vi "Test AO.vi"() -> ()   [LabVIEW 2009, in "MicroDAQ.lvlib"]
uses:
  <instrlib>/MicroDAQ/MicroDAQ.lvlib
  <instrlib>/MicroDAQ/Temp Tests/Test AO enum.ctl
  <instrlib>/MicroDAQ/Tools/Analog mode.ctl
  <instrlib>/MicroDAQ/Tools/Analog Channel Enum.ctl
  <instrlib>/MicroDAQ/Tools/Analo Range Enum.ctl
  <instrlib>/MicroDAQ/Channel/Analog Output/Write NChan NSamp 2D SGL.vi
  <instrlib>/MicroDAQ/Channel/Analog Output/AO Configure Channel.vi
  <instrlib>/MicroDAQ/Channel/Analog Output/Analog output.lvclass
  <instrlib>/MicroDAQ/Channel/Analog Output/Write 1Chan 1Sample SGL.vi
  <instrlib>/MicroDAQ/Channel/Analog Output/Write NChan 1Sample 1D SGL.vi
  <instrlib>/MicroDAQ/MLink32.dll
panel:
  out "Current Test":T1
  in  "Test to execute":T1[](array[typedef])=[enum."Default Config Write NChan NSamp", enum."Default Config Write 1Chan 1Sample", enum."Default Config Write 1Chan 1Sample (with Start)"]
  out "error occured":errorcluster
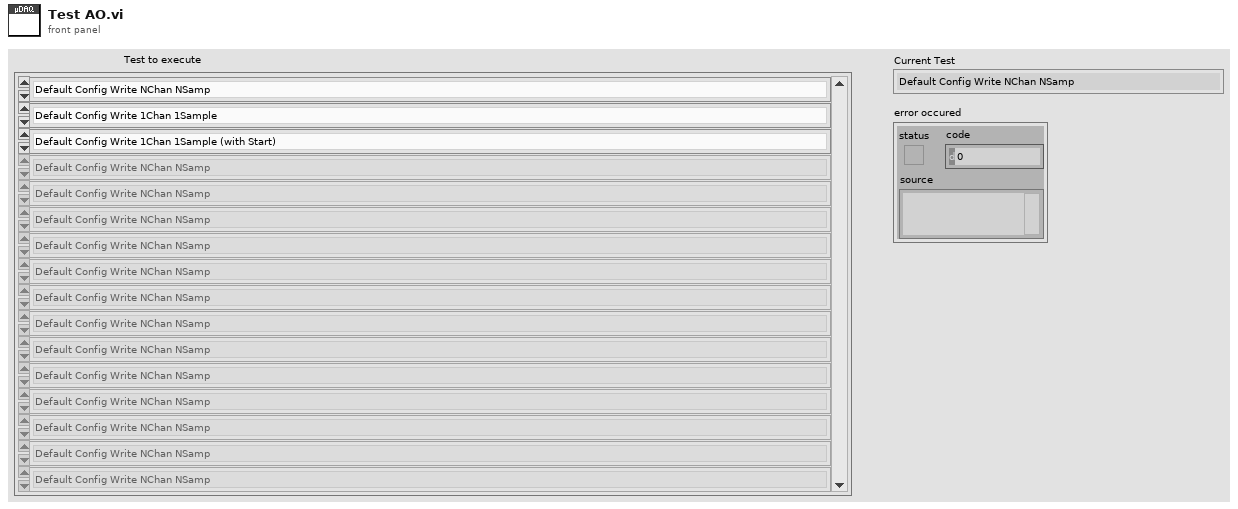
[diagram p1: front panel]
types:
  T1 = typedef "MicroDAQ.lvlib/Test AO enum.ctl" = enum16{"Default Config Write NChan NSamp", "Default Config Write 1Chan 1Sample", "Default Config Write 1Chan 1Sample (with Start)", "Default Config 2Chan NSamp followed by Write 1Samp", "Default Config 2Chan NSamp followed by Write 1Samp followed by Write NSamp"}
  T2 = typedef "MicroDAQ.lvlib/Analog mode.ctl" = enum16{"Periodic", "Stream"}
  T3 = typedef "MicroDAQ.lvlib/Analog Channel Enum.ctl" = enum16{"None", "AO1", "AO2", "AO3", "AO4", "AO5", "AO6", "AO7", "AO8", "AO9", "AO10", "AO11", "AO12", "AO13", "AO14", "AO15", "AO16"}
  T4 = typedef "MicroDAQ.lvlib/Analo Range Enum.ctl" = enum16{"±10V", "0-10V", "±5V", "0-5V", "±5.12V", "±2.56V", "±2.5V", "±2V", "±1.24V", "±0.64V"}
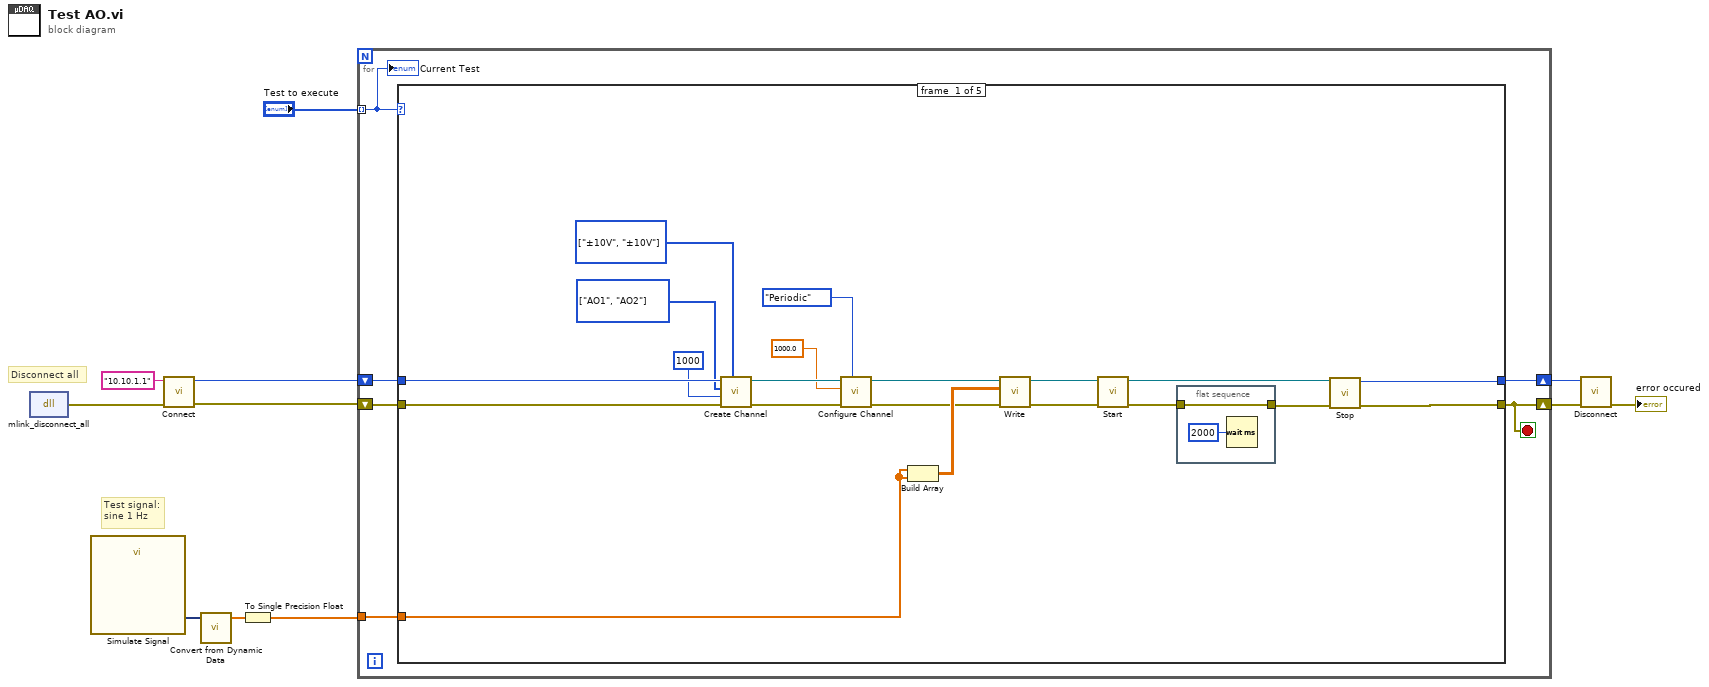
[diagram p0: block diagram]
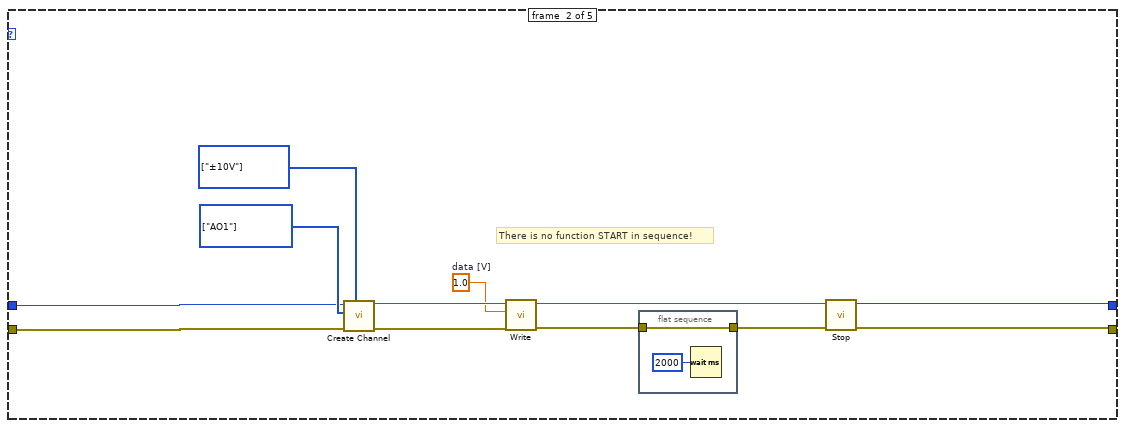
[diagram p2: hidden frame]
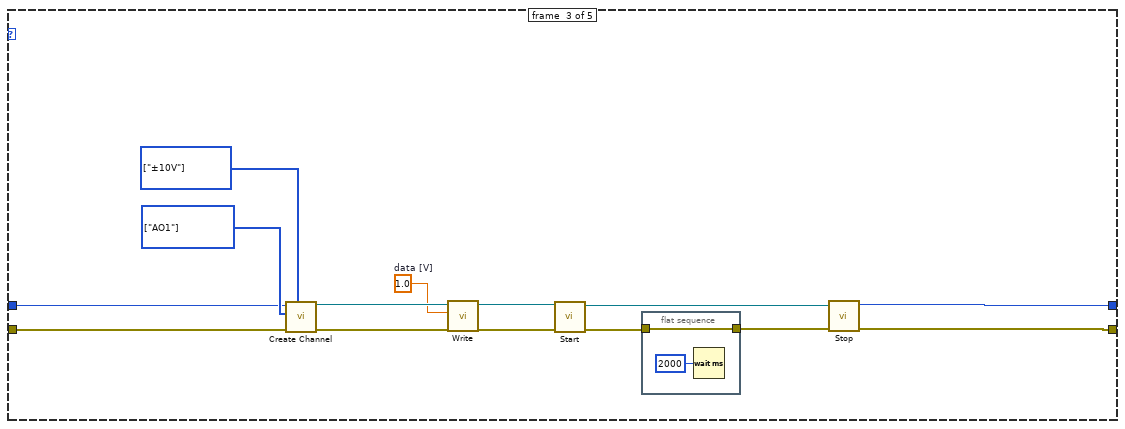
[diagram p3: hidden frame]
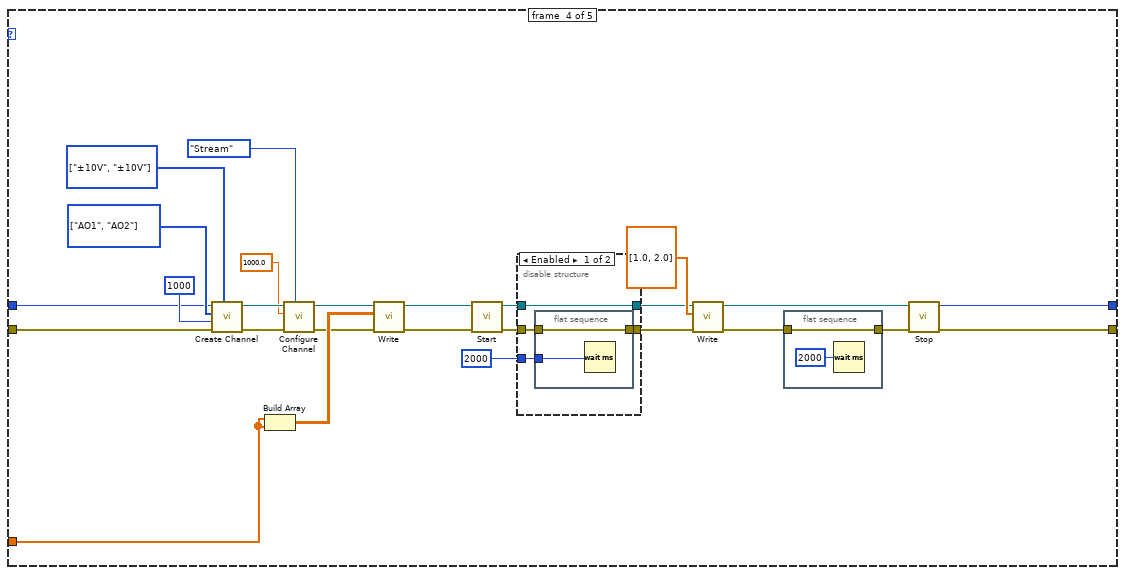
[diagram p4: hidden frame]
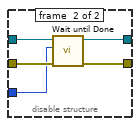
[diagram p5: hidden frame]
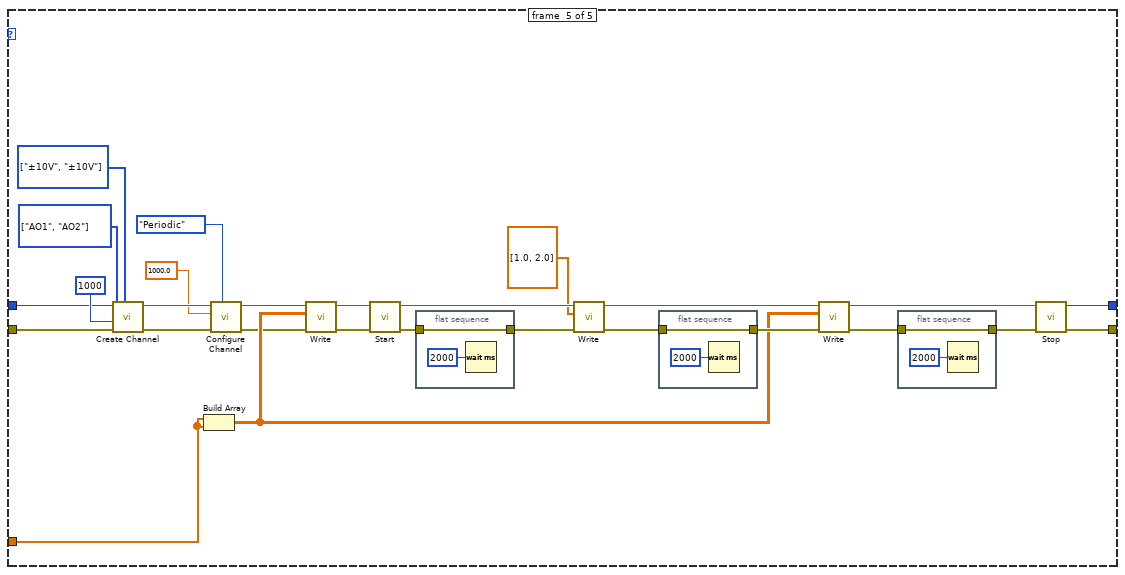
[diagram p6: hidden frame]
diagram:
  # "Test signal:\nsine 1 Hz"
  # "Disconnect all"
  n1 = dll-call lib="C:/Program Files (x86)/National Instruments/LabVIEW 2009/instr.lib/MicroDAQ/MLink32.dll" fn="mlink_disconnect_all" ("MLink32.*:mlink_connect")() -> (error out=w11:errorcluster)  [unwired: 4 in, 1 out]
  n2 = call "Simulate Signal"() -> ("Sine"=w7:dynamicdata)  [unwired: 14 in, 1 out]
  n3 = call <instrlib>:"Connect.vi"("error in (no error)"=w11, "IP address"="10.10.1.1") -> ("error out"=w9:errorcluster, "connection ID"=w10:i32)  [unwired: 8 in]
  n4 = call "Convert from Dynamic Data"("Dynamic Data Type"=w7) -> ("Array"=w6:dbl[])  [unwired: 3 in]
  n5 = To Single Precision Float(number=w6) -> (single precision float=w5:sgl[])
  n6 = for {
    tunnel: w5 -> [w15]
    tunnel: "Test to execute" -> [w14] mode=indexing
    shift-right: [w13] -> w3
    shift-left: w10 -> [w17]
    shift-right: [w12] -> w2
    shift-left: w9 -> [w16]
    stop <- w12 stop-if-true
    n7 = case shown="\"Default Config 2Chan NSamp followed by Write 1Samp followed by Write NSamp\"" w14 {
      tunnel: w17 -> [w37 w49 w61 w80 w125]
      tunnel: w16 -> [w36 w48 w60 w79 w124]
      tunnel: w15 -> [w31 _ _ w83 w123]
      tunnel: [w25 w41 w58 w85 w118] -> w12
      tunnel: [w24 w40 w59 w84 w119] -> w13
      frame #0 {
        w34 = T3[] [enum."AO1", enum."AO2"] items=["None", "AO1", "AO2", "AO3", "AO4", "AO5", "AO6", "AO7", "AO8", "AO9", "AO10", "AO11", "AO12", "AO13", "AO14", "AO15", "AO16"] ("channels")
        w35 = T4[] [enum."±10V", enum."±10V"] items=["±10V", "0-10V", "±5V", "0-5V", "±5.12V", "±2.56V", "±2.5V", "±2V", "±1.24V", "±0.64V"] ("ranges")
        # "AO Basic Config Write (2s) test, 2 Channels"
        n8 = call-poly <instrlib>:"Create Channel.vi"("Ranges"=w35, "error in (no error)"=w36, "Buffer size"=1000 ("buffor size"), "Phisical channels"=w34, "Connection ID"=w37) -> ("error out"=w21:errorcluster, "Task Out"=w23:refnum<class "Analog output.lvclass">)  [unwired: 5 in]
        n9 = call-poly <instrlib>:"Configure Channel.vi"("Mode"=Analog_mode."Periodic", "error in (no error)"=w21, "Sample rate"=1000.0, "Analog Output in"=w23) -> ("error out"=w20:errorcluster, "Analog Output out"=w19:refnum<class "Analog output.lvclass">)  [unwired: 6 in]
        n10 = Build Array(w31, w31) -> (w32:sgl[][])
        n11 = call-poly <instrlib>:"Write.vi"("error in (no error)"=w20, "data"=w32, "Analog Output in"=w19) -> ("error out"=w29:errorcluster, "Analog Output out"=w30:refnum<class "Analog output.lvclass">)  [unwired: 7 in]
        n12 = call-dynamic "Start.vi"("error in (no error)"=w29, "Analog Output in"=w30) -> ("error out"=w28:errorcluster, "Analog Output out"=w26:refnum<class "Analog output.lvclass">)  [unwired: 8 in]
        n13 = flat-sequence {
          tunnel: w28 -> [w38]
          tunnel: [w38] -> w27
          frame #0 {
            n14 = Wait (ms)(milliseconds to wait=u32 2000) -> ()  [unwired: 1 out]
          }
        }
        n15 = call-dynamic "Stop.vi"("error in (no error)"=w27, "Analog Output in"=w26) -> ("error out"=w25:errorcluster, "connection ID"=w24:i32)  [unwired: 8 in]
      }
      frame #1 {
        w45 = sgl 1.0  # data [V]
        w50 = T3[] [enum."AO1"] items=["None", "AO1", "AO2", "AO3", "AO4", "AO5", "AO6", "AO7", "AO8", "AO9", "AO10", "AO11", "AO12", "AO13", "AO14", "AO15", "AO16"] ("channels")
        w51 = T4[] [enum."±10V"] items=["±10V", "0-10V", "±5V", "0-5V", "±5.12V", "±2.56V", "±2.5V", "±2V", "±1.24V", "±0.64V"] ("ranges")
        # "There is no function START in sequence!"
        n16 = call-poly <instrlib>:"Create Channel.vi"("Ranges"=w51, "error in (no error)"=w48, "Phisical channels"=w50, "Connection ID"=w49) -> ("error out"=w46:errorcluster, "Task Out"=w47:refnum<class "Analog output.lvclass">)  [unwired: 6 in]
        n17 = call-poly <instrlib>:"Write.vi"("error in (no error)"=w46, "data"=w45, "Analog Output in"=w47) -> ("error out"=w43:errorcluster, "Analog Output out"=w44:refnum<class "Analog output.lvclass">)  [unwired: 7 in]
        n18 = flat-sequence {
          tunnel: w43 -> [w52]
          tunnel: [w52] -> w42
          frame #0 {
            n19 = Wait (ms)(milliseconds to wait=u32 2000) -> ()  [unwired: 1 out]
          }
        }
        n20 = call-dynamic "Stop.vi"("error in (no error)"=w42, "Analog Output in"=w44) -> ("error out"=w41:errorcluster, "connection ID"=w40:i32)  [unwired: 8 in]
      }
      frame #2 {
        w63 = sgl 1.0  # data [V]
        w66 = T3[] [enum."AO1"] items=["None", "AO1", "AO2", "AO3", "AO4", "AO5", "AO6", "AO7", "AO8", "AO9", "AO10", "AO11", "AO12", "AO13", "AO14", "AO15", "AO16"] ("channels")
        w67 = T4[] [enum."±10V"] items=["±10V", "0-10V", "±5V", "0-5V", "±5.12V", "±2.56V", "±2.5V", "±2V", "±1.24V", "±0.64V"] ("ranges")
        n21 = call-poly <instrlib>:"Create Channel.vi"("Ranges"=w67, "error in (no error)"=w60, "Phisical channels"=w66, "Connection ID"=w61) -> ("error out"=w64:errorcluster, "Task Out"=w65:refnum<class "Analog output.lvclass">)  [unwired: 6 in]
        n22 = call-poly <instrlib>:"Write.vi"("error in (no error)"=w64, "data"=w63, "Analog Output in"=w65) -> ("error out"=w57:errorcluster, "Analog Output out"=w56:refnum<class "Analog output.lvclass">)  [unwired: 7 in]
        n23 = call-dynamic "Start.vi"("error in (no error)"=w57, "Analog Output in"=w56) -> ("error out"=w54:errorcluster, "Analog Output out"=w55:refnum<class "Analog output.lvclass">)  [unwired: 8 in]
        n24 = flat-sequence {
          tunnel: w54 -> [w68]
          tunnel: [w68] -> w62
          frame #0 {
            n25 = Wait (ms)(milliseconds to wait=u32 2000) -> ()  [unwired: 1 out]
          }
        }
        n26 = call-dynamic "Stop.vi"("error in (no error)"=w62, "Analog Output in"=w55) -> ("error out"=w58:errorcluster, "connection ID"=w59:i32)  [unwired: 8 in]
      }
      frame #3 {
        w94 = T3[] [enum."AO1", enum."AO2"] items=["None", "AO1", "AO2", "AO3", "AO4", "AO5", "AO6", "AO7", "AO8", "AO9", "AO10", "AO11", "AO12", "AO13", "AO14", "AO15", "AO16"] ("channels")
        w95 = T4[] [enum."±10V", enum."±10V"] items=["±10V", "0-10V", "±5V", "0-5V", "±5.12V", "±2.56V", "±2.5V", "±2V", "±1.24V", "±0.64V"] ("ranges")
        n27 = call-poly <instrlib>:"Create Channel.vi"("Ranges"=w95, "error in (no error)"=w79, "Buffer size"=1000 ("buffor size"), "Phisical channels"=w94, "Connection ID"=w80) -> ("error out"=w77:errorcluster, "Task Out"=w78:refnum<class "Analog output.lvclass">)  [unwired: 5 in]
        n28 = Build Array(w83, w83) -> (w82:sgl[][])
        n29 = call-poly <instrlib>:"Configure Channel.vi"("Mode"=Analog_mode."Stream", "error in (no error)"=w77, "Sample rate"=1000.0, "Analog Output in"=w78) -> ("error out"=w76:errorcluster, "Analog Output out"=w75:refnum<class "Analog output.lvclass">)  [unwired: 6 in]
        n30 = call-poly <instrlib>:"Write.vi"("error in (no error)"=w76, "data"=w82, "Analog Output in"=w75) -> ("error out"=w91:errorcluster, "Analog Output out"=w92:refnum<class "Analog output.lvclass">)  [unwired: 7 in]
        n31 = call-dynamic "Start.vi"("error in (no error)"=w91, "Analog Output in"=w92) -> ("error out"=w90:errorcluster, "Analog Output out"=w73:refnum<class "Analog output.lvclass">)  [unwired: 8 in]
        n32 = disable-structure shown="Enabled" {
          disable-tunnel: w90 -> [w99 w106]
          disable-tunnel: [w98 w103] -> w89
          disable-tunnel: w73 -> [w97 w105]
          disable-tunnel: [w97 w104] -> w72
          disable-tunnel: u32 2000 ("milliseconds to wait") -> [w96 w102]
          frame #0 {
            n33 = flat-sequence {
              tunnel: w99 -> [w101]
              tunnel: [w101] -> w98
              tunnel: w96 -> [w100]
              frame #0 {
                n34 = Wait (ms)(milliseconds to wait=w100) -> ()  [unwired: 1 out]
              }
            }
          }
          frame #1 {
            n35 = call-dynamic "Wait until Done.vi"("error in (no error)"=w106, "timeout [s]"=w102, "Analog output in"=w105) -> ("error out"=w103:errorcluster, "Analog output out"=w104:refnum<class "Analog output.lvclass">)  [unwired: 7 in]
          }
        }
        n36 = call-poly <instrlib>:"Write.vi"("error in (no error)"=w89, "data"=dbl[] [1.0, 2.0], "Analog Output in"=w72) -> ("error out"=w88:errorcluster, "Analog Output out"=w87:refnum<class "Analog output.lvclass">)  [unwired: 7 in]
        n37 = flat-sequence {
          tunnel: w88 -> [w107]
          tunnel: [w107] -> w86
          frame #0 {
            n38 = Wait (ms)(milliseconds to wait=u32 2000) -> ()  [unwired: 1 out]
          }
        }
        n39 = call-dynamic "Stop.vi"("error in (no error)"=w86, "Analog Output in"=w87) -> ("error out"=w85:errorcluster, "connection ID"=w84:i32)  [unwired: 8 in]
      }
      frame #4 {
        w134 = T3[] [enum."AO1", enum."AO2"] items=["None", "AO1", "AO2", "AO3", "AO4", "AO5", "AO6", "AO7", "AO8", "AO9", "AO10", "AO11", "AO12", "AO13", "AO14", "AO15", "AO16"] ("channels")
        w135 = T4[] [enum."±10V", enum."±10V"] items=["±10V", "0-10V", "±5V", "0-5V", "±5.12V", "±2.56V", "±2.5V", "±2V", "±1.24V", "±0.64V"] ("ranges")
        n40 = call-poly <instrlib>:"Create Channel.vi"("Ranges"=w135, "error in (no error)"=w124, "Buffer size"=1000 ("buffor size"), "Phisical channels"=w134, "Connection ID"=w125) -> ("error out"=w113:errorcluster, "Task Out"=w114:refnum<class "Analog output.lvclass">)  [unwired: 5 in]
        n41 = Build Array(w123, w123) -> (w117:sgl[][])
        n42 = call-poly <instrlib>:"Configure Channel.vi"("Mode"=Analog_mode."Periodic", "error in (no error)"=w113, "Sample rate"=1000.0, "Analog Output in"=w114) -> ("error out"=w112:errorcluster, "Analog Output out"=w111:refnum<class "Analog output.lvclass">)  [unwired: 6 in]
        n43 = call-poly <instrlib>:"Write.vi"("error in (no error)"=w112, "data"=w117, "Analog Output in"=w111) -> ("error out"=w131:errorcluster, "Analog Output out"=w132:refnum<class "Analog output.lvclass">)  [unwired: 7 in]
        n44 = call-dynamic "Start.vi"("error in (no error)"=w131, "Analog Output in"=w132) -> ("error out"=w130:errorcluster, "Analog Output out"=w127:refnum<class "Analog output.lvclass">)  [unwired: 8 in]
        n45 = flat-sequence {
          tunnel: w130 -> [w140]
          tunnel: [w140] -> w129
          frame #0 {
            n46 = Wait (ms)(milliseconds to wait=u32 2000) -> ()  [unwired: 1 out]
          }
        }
        n47 = call-poly <instrlib>:"Write.vi"("error in (no error)"=w129, "data"=sgl[] [1.0, 2.0], "Analog Output in"=w127) -> ("error out"=w128:errorcluster, "Analog Output out"=w122:refnum<class "Analog output.lvclass">)  [unwired: 7 in]
        n48 = flat-sequence {
          tunnel: w128 -> [w138]
          tunnel: [w138] -> w121
          frame #0 {
            n49 = Wait (ms)(milliseconds to wait=u32 2000) -> ()  [unwired: 1 out]
          }
        }
        n50 = call-poly <instrlib>:"Write.vi"("error in (no error)"=w121, "data"=w117, "Analog Output in"=w122) -> ("error out"=w116:errorcluster, "Analog Output out"=w120:refnum<class "Analog output.lvclass">)  [unwired: 7 in]
        n51 = flat-sequence {
          tunnel: w116 -> [w136]
          tunnel: [w136] -> w115
          frame #0 {
            n52 = Wait (ms)(milliseconds to wait=u32 2000) -> ()  [unwired: 1 out]
          }
        }
        n53 = call-dynamic "Stop.vi"("error in (no error)"=w115, "Analog Output in"=w120) -> ("error out"=w118:errorcluster, "connection ID"=w119:i32)  [unwired: 8 in]
      }
    }
    "Current Test" <- w14
  }
  n54 = call <instrlib>:"Disconnect.vi"("error in (no error)"=w2, "connection ID"=w3) -> ("error out"=→"error occured":errorcluster)  [unwired: 9 in]
